vi "Zaber A Series Control Panel.vi"() -> ()   [LabVIEW 2012]
doc: "This VI is a control panel that allows the user to perform a variety of commands and motions, see what devices are connected, read and change settings and track the movements, It is both an example of the way you can use the instrument library as well as a versatile tool for everyday usage."
uses:
  <instrlib>/Zaber A Series/Zaber A Series.lvlib
panel:
  in  "Data":string
  in  "Command List":string(combo)="get"
  in  "Units (0: microsteps)":u16(ring) items=["microsteps", "microns", "millimeters", "inches"]
  in  "Movement Type (0: relative)":u16(ring) items=["relative", "absolute"]
  in  "Home":bool
  out "Command Responses":string[](array[string])
  out "Device Information":string[][](array[string])
  in  "Identify Devices":bool
  in  "Device Number & Axis":string(combo)
  in  "Start Tracking":bool
  out "Position":dbl
  out "Current Value":string
  in  "Execute Movement":bool
  in  "Move Distance (0)":dbl
  in  "Microstep Size (0)":dbl
  in  "Send Command":bool
  in  "Value to Send":string
  in  "Change Setting":bool
  in  "Get Setting":bool
  in  "Setting":string(combo)
  in  "VISA resource name":refnum<visa-resource-name>
  in  "Close Port":bool
  in  "Open Port":bool
  in  "Quit":bool
  # "For information on what each function panel does, how the VI works, and example usages of the library VIs see the notes in the Block Diagram and the library VI help descriptions. Email contact@zaber.com for any questions on usage."
  # "Zaber ASCII Control Panel"
  # "(c) 2014 Zaber Technologies.  ALL RIGHTS RESERVED."
  # "Port Settings"
  # "Shared Settings"
  # "Position Tracking"
  # "Read and Modify Settings"
  # "Send Command"
  # "Identify Connected Devices"
  # "Send Movement"
  # "Device Number"
  # "Model Name"
  # "Microstep Size (um)"
  # "Home Devices"
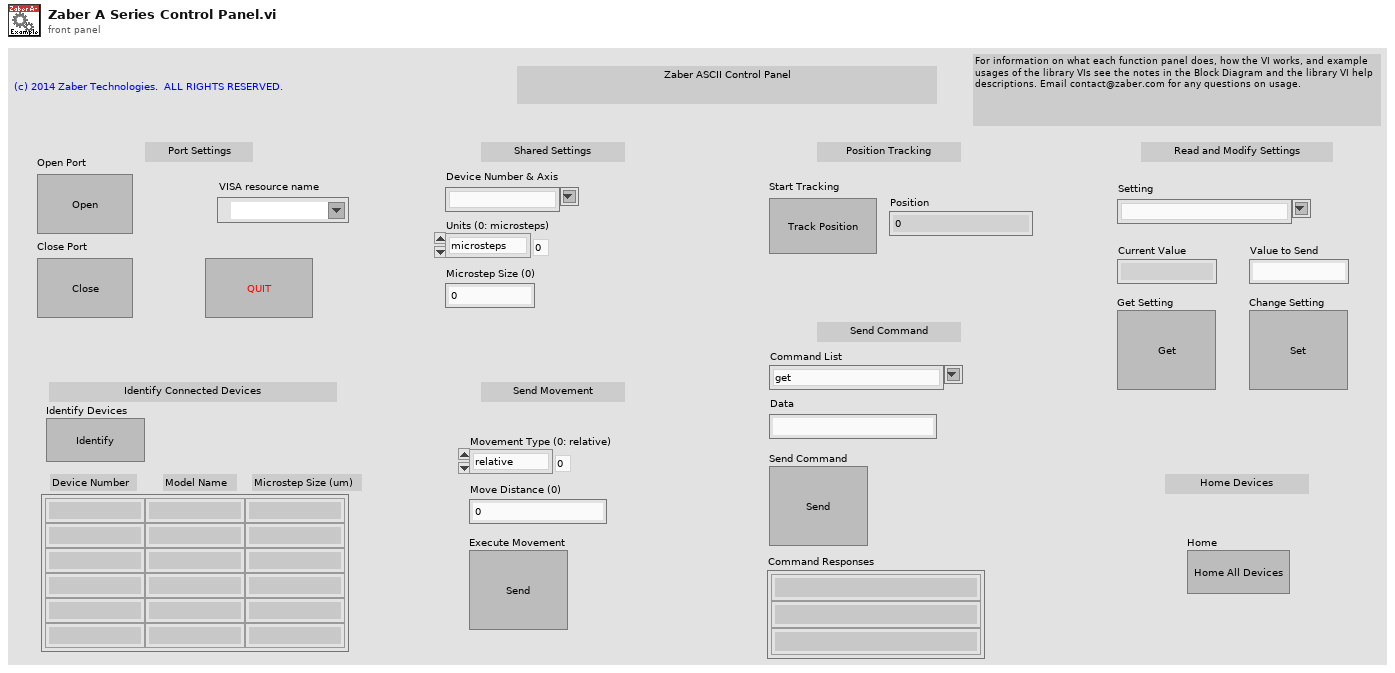
[diagram p1: front panel]
types:
  T1 = enum8{"Enabled", "Disabled", "Disabled and Grayed Out"}
  T2 = cluster{"Device":string, "Axis":string, "Reply Flag":string, "Status":string, "Warning Flags":string, "Data":string}[]
  T3 = cluster{"Device":string, "Axis":string, "Reply Flag":string, "Status":string, "Warning Flags":string, "Data":string}
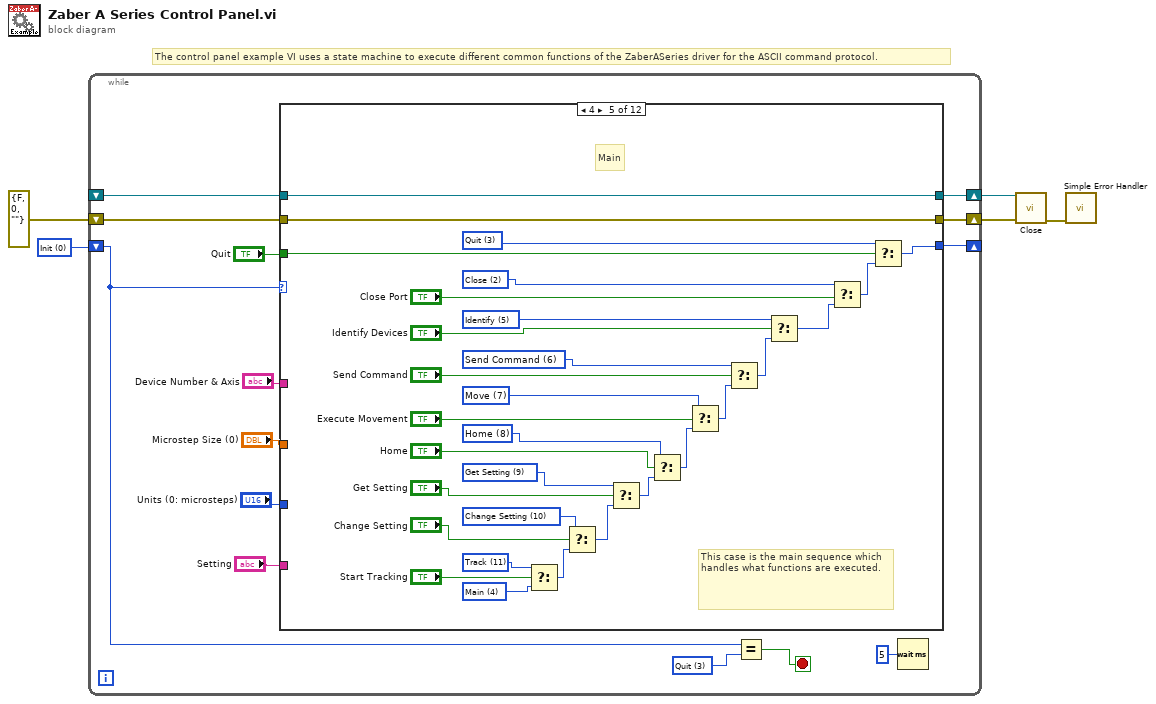
[diagram p0: block diagram]
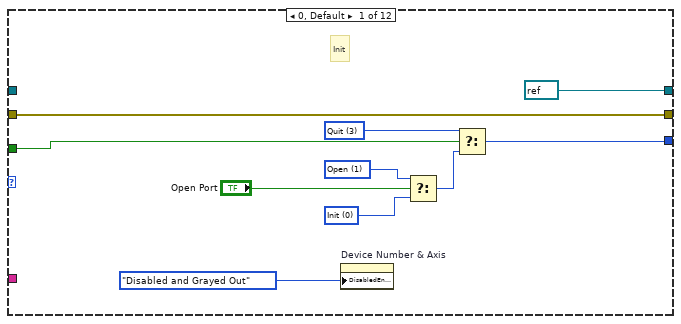
[diagram p2: hidden frame]
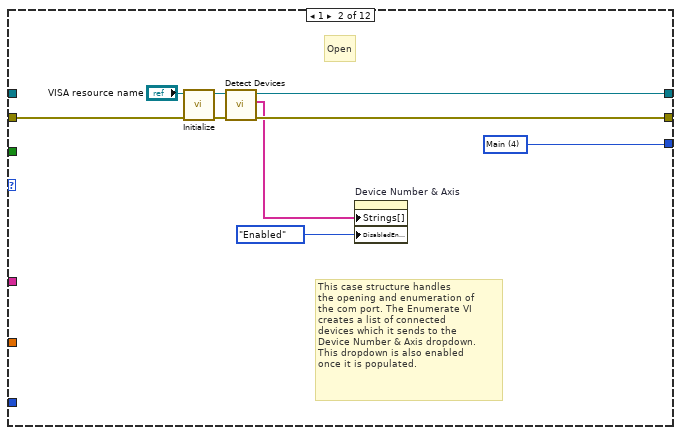
[diagram p3: hidden frame]
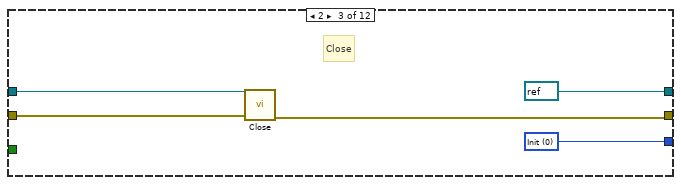
[diagram p4: hidden frame]
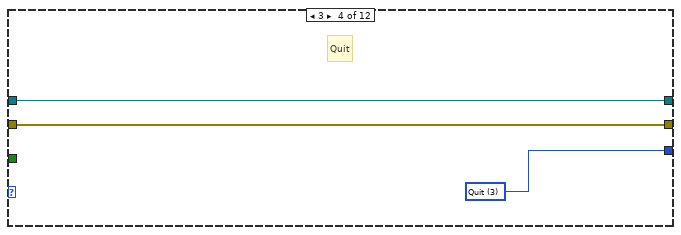
[diagram p5: hidden frame]
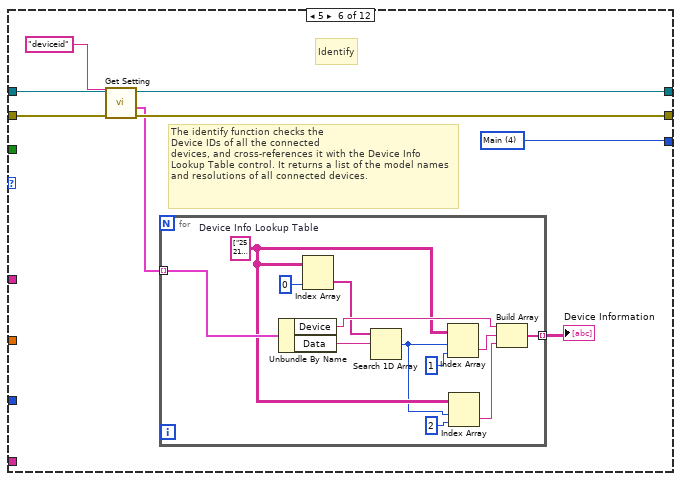
[diagram p6: hidden frame]
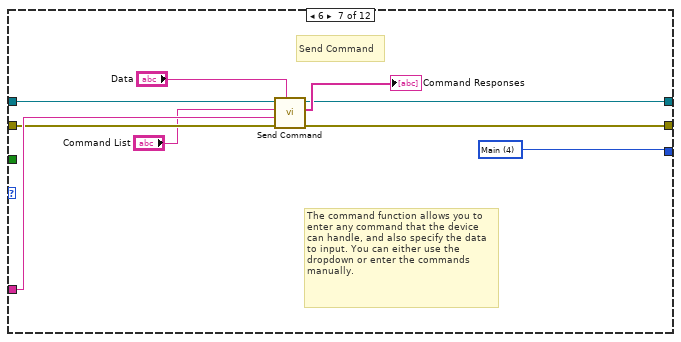
[diagram p7: hidden frame]
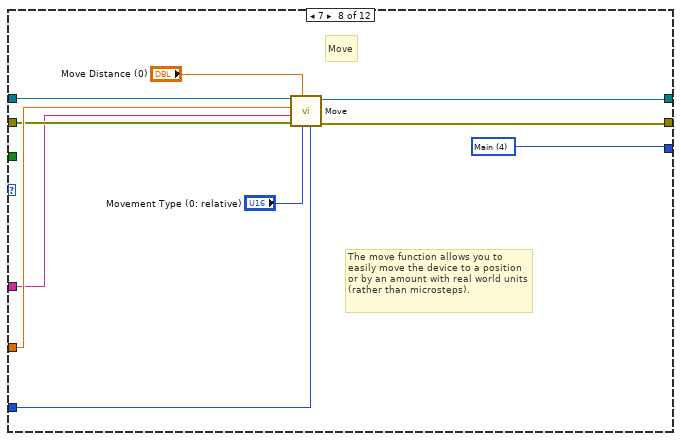
[diagram p8: hidden frame]
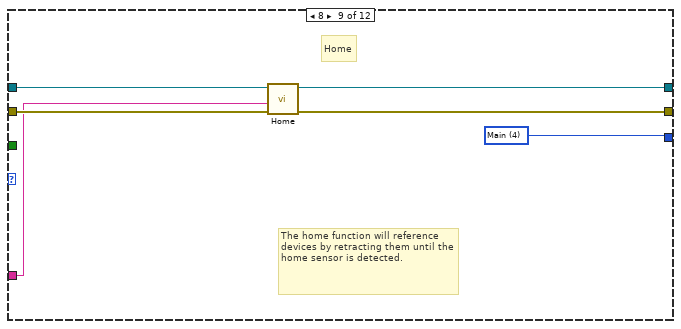
[diagram p9: hidden frame]
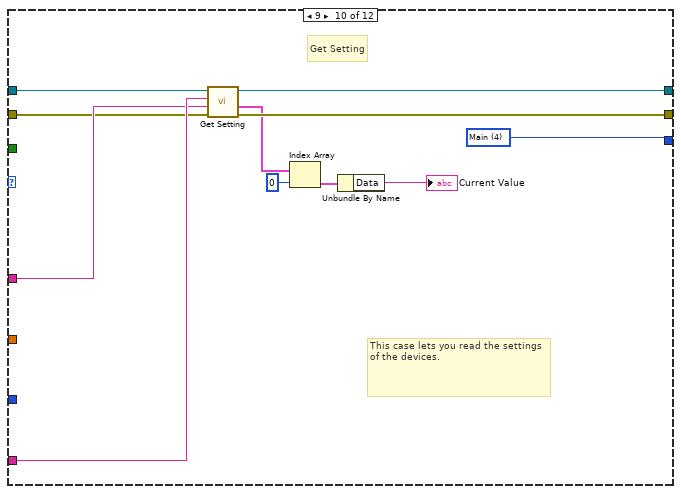
[diagram p10: hidden frame]
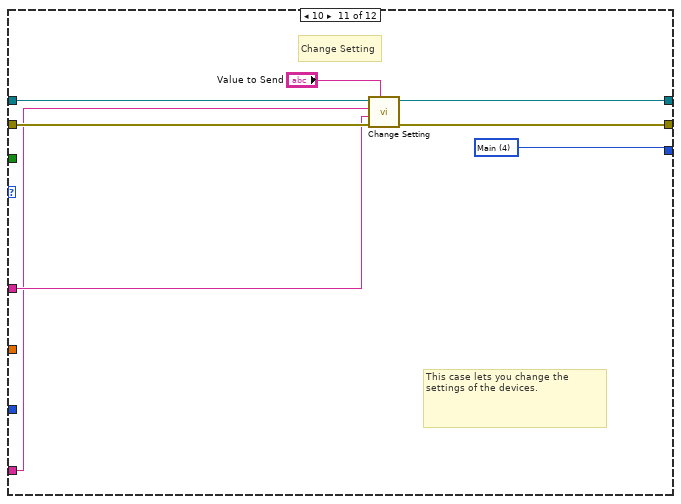
[diagram p11: hidden frame]
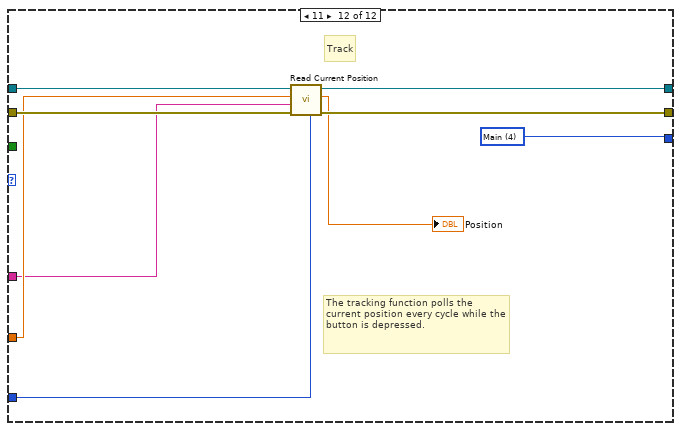
[diagram p12: hidden frame]
diagram:
  w5 = u16 0 items=["Init", "Open", "Close", "Quit", "Main", "Identify", "Send Command", "Move", "Home", "Get Setting", "Change Setting", "Track"]
  # "The control panel example VI uses a state machine to execute different common functions of the ZaberASeries driver for the ASCII command protocol."
  n1 = while {
    shift-right: [w16] -> _
    shift-left: w5 -> [w18]
    shift-right: [w14] -> w3
    shift-left: _ -> [w13]
    shift-right: [w8] -> w2
    shift-left: errorcluster {"status"=FALSE, "code"=0, "source"=""} ("error out") -> [w7]
    stop <- w19 stop-if-true
    w17 = u16 3 items=["Init", "Open", "Close", "Quit", "Main", "Identify", "Send Command", "Move", "Home", "Get Setting", "Change Setting", "Track"]
    n2 = case shown="4" w18 {
      tunnel: [w25 w38 w39 w46 w48 w84 w105 w115 w121 w132 w140 w149] -> w16
      tunnel: "Quit" -> [w29 _ _ _ w50 _ _ _ _ _ _ _]
      tunnel: [refnum<visa-resource-name> refnum ("VISA resource name") w34 refnum<visa-resource-name> refnum ("VISA resource name out") w45 w56 w79 w99 w108 w118 w122 w139 w147] -> w14
      tunnel: w13 -> [_ _ w42 w45 w56 w82 w104 w110 w120 w127 w138 w148]
      tunnel: "Setting" -> [_ _ _ _ _ _ _ _ _ w128 w133 _]
      tunnel: "Units (0: microsteps)" -> [_ _ _ _ _ _ _ w112 _ _ _ w143]
      tunnel: "Microstep Size (0)" -> [_ _ _ _ _ _ _ w111 _ _ _ w142]
      tunnel: "Device Number & Axis" -> [_ _ _ _ _ _ w103 w106 w116 w126 w135 w141]
      tunnel: [w20 w32 w40 w44 w55 w80 w101 w107 w117 w124 w136 w145] -> w8
      tunnel: w7 -> [w20 w31 w41 w44 w55 w81 w102 w109 w119 w125 w137 w146]
      frame 0, Default {
        w23 = u16 0 items=["Init", "Open", "Close", "Quit", "Main", "Identify", "Send Command", "Move", "Home", "Get Setting", "Change Setting", "Track"]
        w24 = u16 1 items=["Init", "Open", "Close", "Quit", "Main", "Identify", "Send Command", "Move", "Home", "Get Setting", "Change Setting", "Track"]
        w27 = u16 3 items=["Init", "Open", "Close", "Quit", "Main", "Identify", "Send Command", "Move", "Home", "Get Setting", "Change Setting", "Track"]
        # "Init"
        n3 = property on="Device Number & Axis" class="CmbBox"("DisabledEnum"=T1."Disabled and Grayed Out" ("Disabled")) -> ()  [unwired: 2 in, 2 out]
        n4 = Select(t=w24, s="Open Port", f=w23) -> (s? t:f=w26:u16)
        n5 = Select(t=w27, s=w29, f=w26) -> (s? t:f=w25:u16)
      }
      frame 1 {
        w38 = u16 4 items=["Init", "Open", "Close", "Quit", "Main", "Identify", "Send Command", "Move", "Home", "Get Setting", "Change Setting", "Track"]
        # "This case structure handles \nthe opening and enumeration of\nthe com port. The Enumerate VI \ncreates a list of connected\ndevices which it sends to the\nDevice Number & Axis dropdown. \nThis dropdown is also enabled\nonce it is populated."
        # "Open"
        n6 = call <instrlib>:"Initialize.vi"("error in (no error)"=w31, "VISA resource name"="VISA resource name") -> ("error out"=w33:errorcluster, "VISA resource name out"=w35:refnum<visa-resource-name>)  [unwired: 8 in]
        n7 = call <instrlib>:"Detect Devices.vi"("error in (no error)"=w33, "VISA resource name"=w35) -> ("error out"=w32:errorcluster, "Connected Devices and Axes"=w30:string[], "VISA resource name out"=w34:refnum<visa-resource-name>)  [unwired: 7 in]
        n8 = property on="Device Number & Axis" class="CmbBox"("Strings[]"=w30, "DisabledEnum"=T1."Enabled" ("Disabled")) -> ()  [unwired: 2 in, 2 out]
      }
      frame 2 {
        w39 = u16 0 items=["Init", "Open", "Close", "Quit", "Main", "Identify", "Send Command", "Move", "Home", "Get Setting", "Change Setting", "Track"]
        # "Close"
        n9 = call <instrlib>:"Close.vi"("error in (no error)"=w41, "VISA resource name"=w42) -> ("error out"=w40:errorcluster)  [unwired: 9 in]
      }
      frame 3 {
        w46 = u16 3 items=["Init", "Open", "Close", "Quit", "Main", "Identify", "Send Command", "Move", "Home", "Get Setting", "Change Setting", "Track"]
        # "Quit"
      }
      frame 4 {
        w47 = u16 3 items=["Init", "Open", "Close", "Quit", "Main", "Identify", "Send Command", "Move", "Home", "Get Setting", "Change Setting", "Track"]
        w52 = u16 2 items=["Init", "Open", "Close", "Quit", "Main", "Identify", "Send Command", "Move", "Home", "Get Setting", "Change Setting", "Track"]
        w53 = u16 4 items=["Init", "Open", "Close", "Quit", "Main", "Identify", "Send Command", "Move", "Home", "Get Setting", "Change Setting", "Track"]
        w70 = u16 11 items=["Init", "Open", "Close", "Quit", "Main", "Identify", "Send Command", "Move", "Home", "Get Setting", "Change Setting", "Track"]
        w71 = u16 10 items=["Init", "Open", "Close", "Quit", "Main", "Identify", "Send Command", "Move", "Home", "Get Setting", "Change Setting", "Track"]
        w72 = u16 9 items=["Init", "Open", "Close", "Quit", "Main", "Identify", "Send Command", "Move", "Home", "Get Setting", "Change Setting", "Track"]
        w73 = u16 8 items=["Init", "Open", "Close", "Quit", "Main", "Identify", "Send Command", "Move", "Home", "Get Setting", "Change Setting", "Track"]
        w74 = u16 7 items=["Init", "Open", "Close", "Quit", "Main", "Identify", "Send Command", "Move", "Home", "Get Setting", "Change Setting", "Track"]
        w76 = u16 6 items=["Init", "Open", "Close", "Quit", "Main", "Identify", "Send Command", "Move", "Home", "Get Setting", "Change Setting", "Track"]
        w75 = u16 5 items=["Init", "Open", "Close", "Quit", "Main", "Identify", "Send Command", "Move", "Home", "Get Setting", "Change Setting", "Track"]
        # "This case is the main sequence which handles what functions are executed."
        # "Main"
        n10 = Select(t=w70, s="Start Tracking", f=w53) -> (s? t:f=w69:u16)
        n11 = Select(t=w71, s="Change Setting", f=w69) -> (s? t:f=w68:u16)
        n12 = Select(t=w72, s="Get Setting", f=w68) -> (s? t:f=w67:u16)
        n13 = Select(t=w73, s="Home", f=w67) -> (s? t:f=w66:u16)
        n14 = Select(t=w74, s="Execute Movement", f=w66) -> (s? t:f=w65:u16)
        n15 = Select(t=w76, s="Send Command", f=w65) -> (s? t:f=w64:u16)
        n16 = Select(t=w75, s="Identify Devices", f=w64) -> (s? t:f=w54:u16)
        n17 = Select(t=w52, s="Close Port", f=w54) -> (s? t:f=w49:u16)
        n18 = Select(t=w47, s=w50, f=w49) -> (s? t:f=w48:u16)
      }
      frame 5 {
        w84 = u16 4 items=["Init", "Open", "Close", "Quit", "Main", "Identify", "Send Command", "Move", "Home", "Get Setting", "Change Setting", "Track"]
        # "The identify function checks the\nDevice IDs of all the connected \ndevices, and cross-references it with the Device Info Lookup Table control. It returns a list of the model names and resolutions of all connected devices."
        # "Identify"
        n19 = call <instrlib>:"Get Setting.vi"("error in (no error)"=w81, "Setting"="deviceid" ("Common Settings"), "VISA resource name"=w82) -> ("error out"=w80:errorcluster, "Response Bundle Array"=w77:T2, "VISA resource name out"=w79:refnum<visa-resource-name>)  [unwired: 4 in, 2 out]
        n20 = for {
          tunnel: w77 -> [w96] mode=indexing
          tunnel: [w93] -> w83 mode=indexing
          w91 = string[][] [["25213", "A-BAR200BLC", "0.248046875"], ["25313", "A-BAR200BLC-E01", "0.248046875"], ["25214", "A-BAR300BLC", "0.248046875"], ["25314", "A-BAR300BLC-E01", "0.248046875"], ["22011", "A-BLQ0070", "4.21875"], ["22111", "A-BLQ0070-E01", "4.21875"], ["22112", "A-BLQ0070-E01L", "4.21875"], ["22012", "A-BLQ0070-L", "4.21875"], ["22021", "A-BLQ0145", "4.21875"], ["22121", "A-BLQ0145-E01", "4.21875"], ["22122", "A-BLQ0145-E01L", "4.21875"], ["22022", "A-BLQ0145-L", "4.21875"], ["22031", "A-BLQ0295", "4.21875"], ["22131", "A-BLQ0295-E01", "4.21875"], ["22132", "A-BLQ0295-E01L", "4.21875"], ["22032", "A-BLQ0295-L", "4.21875"], ["22041", "A-BLQ0445", "4.21875"], ["22141", "A-BLQ0445-E01", "4.21875"], ["22142", "A-BLQ0445-E01L", "4.21875"], ["22042", "A-BLQ0445-L", "4.21875"], ["22051", "A-BLQ0595", "4.21875"], ["22151", "A-BLQ0595-E01", "4.21875"], ["22152", "A-BLQ0595-E01L", "4.21875"], ["22052", "A-BLQ0595-L", "4.21875"], ["22061", "A-BLQ1045", "4.21875"], ["22161", "A-BLQ1045-E01", "4.21875"], ["22162", "A-BLQ1045-E01L", "4.21875"], ["22062", "A-BLQ1045-L", "4.21875"], ["22071", "A-BLQ1495", "4.21875"], ["22171", "A-BLQ1495-E01", "4.21875"], ["22172", "A-BLQ1495-E01L", "4.21875"], ["22072", "A-BLQ1495-L", "4.21875"], ["22081", "A-BLQ2095", "4.21875"], ["22181", "A-BLQ2095-E01", "4.21875"], ["22182", "A-BLQ2095-E01L", "4.21875"], ["22082", "A-BLQ2095-L", "4.21875"], ["25011", "A-LAR200ALC", "0.1984375"], ["25111", "A-LAR200ALC-E01", "0.1984375"], ["25012", "A-LAR300ALC", "0.1984375"], ["25112", "A-LAR300ALC-E01", "0.1984375"], ["20011", "A-LSQ075A", "0.09921875"], ["20111", "A-LSQ075A-E01", "0.09921875"], ["20012", "A-LSQ075B", "0.49609375"], ["20112", "A-LSQ075B-E01", "0.49609375"], ["20013", "A-LSQ075D", "1.984375"], ["20113", "A-LSQ075D-E01", "1.984375"], ["20021", "A-LSQ150A", "0.09921875"], ["20121", "A-LSQ150A-E01", "0.09921875"], ["20022", "A-LSQ150B", "0.49609375"], ["20122", "A-LSQ150B-E01", "0.49609375"], ["20023", "A-LSQ150D", "1.984375"], ["20123", "A-LSQ150D-E01", "1.984375"], ["20031", "A-LSQ300A", "0.09921875"], ["20131", "A-LSQ300A-E01", "0.09921875"], ["20032", "A-LSQ300B", "0.49609375"], ["20132", "A-LSQ300B-E01", "0.49609375"], ["20033", "A-LSQ300D", "1.984375"], ["20133", "A-LSQ300D-E01", "1.984375"], ["20041", "A-LSQ450A", "0.09921875"], ["20141", "A-LSQ450A-E01", "0.09921875"], ["20042", "A-LSQ450B", "0.49609375"], ["20142", "A-LSQ450B-E01", "0.49609375"], ["20043", "A-LSQ450D", "1.984375"], ["20143", "A-LSQ450D-E01", "1.984375"], ["20051", "A-LSQ600A", "0.09921875"], ["20151", "A-LSQ600A-E01", "0.09921875"], ["20052", "A-LSQ600B", "0.49609375"], ["20152", "A-LSQ600B-E01", "0.49609375"], ["20053", "A-LSQ600D", "1.984375"], ["20153", "A-LSQ600D-E01", "1.984375"], ["21011", "A-LST0250A", "0.124023438"], ["21211", "A-LST0250A-C", "0.124023438"], ["21111", "A-LST0250A-E01", "0.124023438"], ["21311", "A-LST0250A-E01C", "0.124023438"], ["21012", "A-LST0250B", "0.49609375"], ["21212", "A-LST0250B-C", "0.49609375"], ["21112", "A-LST0250B-E01", "0.49609375"], ["21312", "A-LST0250B-E01C", "0.49609375"], ["21013", "A-LST0250D", "1.984375"], ["21213", "A-LST0250D-C", "1.984375"], ["21113", "A-LST0250D-E01", "1.984375"], ["21313", "A-LST0250D-E01C", "1.984375"], ["21021", "A-LST0500A", "0.124023438"], ["21221", "A-LST0500A-C", "0.124023438"], ["21121", "A-LST0500A-E01", "0.124023438"], ["21321", "A-LST0500A-E01C", "0.124023438"], ["21022", "A-LST0500B", "0.49609375"], ["21222", "A-LST0500B-C", "0.49609375"], ["21122", "A-LST0500B-E01", "0.49609375"], ["21322", "A-LST0500B-E01C", "0.49609375"], ["21023", "A-LST0500D", "1.984375"], ["21223", "A-LST0500D-C", "1.984375"], ["21123", "A-LST0500D-E01", "1.984375"], ["21323", "A-LST0500D-E01C", "1.984375"], ["21031", "A-LST0750A", "0.124023438"], ["21231", "A-LST0750A-C", "0.124023438"], ["21131", "A-LST0750A-E01", "0.124023438"], ["21331", "A-LST0750A-E01C", "0.124023438"], ["21032", "A-LST0750B", "0.49609375"], ["21232", "A-LST0750B-C", "0.49609375"], ["21132", "A-LST0750B-E01", "0.49609375"], ["21332", "A-LST0750B-E01C", "0.49609375"], ["21033", "A-LST0750D", "1.984375"], ["21233", "A-LST0750D-C", "1.984375"], ["21133", "A-LST0750D-E01", "1.984375"], ["21333", "A-LST0750D-E01C", "1.984375"], ["21041", "A-LST1000A", "0.124023438"], ["21241", "A-LST1000A-C", "0.124023438"], ["21141", "A-LST1000A-E01", "0.124023438"], ["21341", "A-LST1000A-E01C", "0.124023438"], ["21042", "A-LST1000B", "0.49609375"], ["21242", "A-LST1000B-C", "0.49609375"], ["21142", "A-LST1000B-E01", "0.49609375"], ["21342", "A-LST1000B-E01C", "0.49609375"], ["21043", "A-LST1000D", "1.984375"], ["21243", "A-LST1000D-C", "1.984375"], ["21143", "A-LST1000D-E01", "1.984375"], ["21343", "A-LST1000D-E01C", "1.984375"], ["21051", "A-LST1500A", "0.124023438"], ["21251", "A-LST1500A-C", "0.124023438"], ["21151", "A-LST1500A-E01", "0.124023438"], ["21351", "A-LST1500A-E01C", "0.124023438"], ["21052", "A-LST1500B", "0.49609375"], ["21252", "A-LST1500B-C", "0.49609375"], ["21152", "A-LST1500B-E01", "0.49609375"], ["21352", "A-LST1500B-E01C", "0.49609375"], ["21053", "A-LST1500D", "1.984375"], ["21253", "A-LST1500D-C", "1.984375"], ["21153", "A-LST1500D-E01", "1.984375"], ["21353", "A-LST1500D-E01C", "1.984375"], ["30111", "A-MCA", "var"], ["30221", "A-MCB2", "var"]]  # Device Info Lookup Table
          n21 = Unbundle By Name(w96) -> ("Device"=w94:string, "Data"=w85:string)
          n22 = Index Array(array=w91, index (col)=0 ("disabled index (col)")) -> (element=w92:string[])  [unwired: 1 in]
          n23 = Search 1D Array(1D array=w92, element=w85) -> (index of element=w90:i32)  [unwired: 1 in]
          n24 = Index Array(array=w91, index (row)=w90, index (col)=1 ("disabled index (col)")) -> (element=w87:string)
          n25 = Index Array(array=w91, index (row)=w90, index (col)=2 ("disabled index (col)")) -> (element=w86:string)
          n26 = Build Array(w94, w87, w86) -> (w93:string[])
        }
        "Device Information" <- w83
      }
      frame 6 {
        w105 = u16 4 items=["Init", "Open", "Close", "Quit", "Main", "Identify", "Send Command", "Move", "Home", "Get Setting", "Change Setting", "Track"]
        # "The command function allows you to enter any command that the device can handle, and also specify the data to input. You can either use the dropdown or enter the commands manually."
        # "Send Command"
        n27 = call <instrlib>:"Send Command.vi"("Data"="Data", "error in (no error)"=w102, "Device and Axis"=w103, "Command"="Command List", "VISA resource name"=w104) -> ("error out"=w101:errorcluster, "Response String Array"=→"Command Responses":string[], "VISA resource name out"=w99:refnum<visa-resource-name>)  [unwired: 2 in, 2 out]
      }
      frame 7 {
        w115 = u16 4 items=["Init", "Open", "Close", "Quit", "Main", "Identify", "Send Command", "Move", "Home", "Get Setting", "Change Setting", "Track"]
        # "The move function allows you to easily move the device to a position or by an amount with real world units (rather than microsteps)."
        # "Move"
        n28 = call <instrlib>:"Move.vi"("Units (0: microsteps)"=w112, "Movement Type (0: relative)"="Movement Type (0: relative)", "Move Distance (0)"="Move Distance (0)", "error in (no error)"=w109, "Device and Axis"=w106, "Microstep Size (0)"=w111, "VISA resource name"=w110) -> ("error out"=w107:errorcluster, "VISA resource name out"=w108:refnum<visa-resource-name>)  [unwired: 3 in]
      }
      frame 8 {
        w121 = u16 4 items=["Init", "Open", "Close", "Quit", "Main", "Identify", "Send Command", "Move", "Home", "Get Setting", "Change Setting", "Track"]
        # "The home function will reference  devices by retracting them until the home sensor is detected."
        # "Home"
        n29 = call <instrlib>:"Home.vi"("error in (no error)"=w119, "Device and Axis"=w116, "VISA resource name"=w120) -> ("error out"=w117:errorcluster, "VISA resource name out"=w118:refnum<visa-resource-name>)  [unwired: 7 in]
      }
      frame 9 {
        w132 = u16 4 items=["Init", "Open", "Close", "Quit", "Main", "Identify", "Send Command", "Move", "Home", "Get Setting", "Change Setting", "Track"]
        # "This case lets you read the settings of the devices."
        # "Get Setting"
        n30 = call <instrlib>:"Get Setting.vi"("error in (no error)"=w125, "Device and Axis"=w126, "Setting"=w128, "VISA resource name"=w127) -> ("error out"=w124:errorcluster, "Response Bundle Array"=w123:T2, "VISA resource name out"=w122:refnum<visa-resource-name>)  [unwired: 3 in, 2 out]
        n31 = Index Array(array=w123, index=0 ("index (row)")) -> (element=w130:T3)
        n32 = Unbundle By Name(w130) -> ("Data"=→"Current Value":string)
      }
      frame 10 {
        w140 = u16 4 items=["Init", "Open", "Close", "Quit", "Main", "Identify", "Send Command", "Move", "Home", "Get Setting", "Change Setting", "Track"]
        # "This case lets you change the settings of the devices."
        # "Change Setting"
        n33 = call <instrlib>:"Change Setting.vi"("Data"="Value to Send", "error in (no error)"=w137, "Device and Axis"=w135, "Setting"=w133, "VISA resource name"=w138) -> ("error out"=w136:errorcluster, "VISA resource name out"=w139:refnum<visa-resource-name>)  [unwired: 5 in]
      }
      frame 11 {
        w149 = u16 4 items=["Init", "Open", "Close", "Quit", "Main", "Identify", "Send Command", "Move", "Home", "Get Setting", "Change Setting", "Track"]
        # "The tracking function polls the current position every cycle while the button is depressed."
        # "Track"
        n34 = call <instrlib>:"Read Current Position.vi"("Units (0: microsteps)"=w143, "error in (no error)"=w146, "Device and Axis"=w141, "Microstep Size (0)"=w142, "VISA resource name"=w148) -> ("error out"=w145:errorcluster, "Position"=→"Position":dbl, "VISA resource name out"=w147:refnum<visa-resource-name>)  [unwired: 4 in]
      }
    }
    n35 = Equal?(x=w18, y=w17) -> (x = y?=w19:bool)
    n36 = Wait (ms)(milliseconds to wait=u32 5) -> ()  [unwired: 1 out]
  }
  n37 = call <instrlib>:"Close.vi"("error in (no error)"=w2, "VISA resource name"=w3) -> ("error out"=w1:errorcluster)  [unwired: 9 in]
  n38 = call <vilib>:"Simple Error Handler.vi"("error in (no error)"=w1) -> ()  [unwired: 4 in, 5 out]
